vi "Insight_WL-OptFreq_Converter.vi"(6 "Units":T1(ring), 8 "error in (no error)":errorcluster, 11 "WL or Opt. Freq":dbl[](array[numeric])) -> (0 "error out":errorcluster, 3 "Opt. Freq or WL":dbl[](array[numeric]))   [LabVIEW 2010]
doc: "Insight Photonic Solutions\n\nThis VI converts wavelength to optical frequency, and vice-versa. Just input one, and the VI produces the other. Select units for wavelength and frequency.\n\nINPUTS\n\nUnits - for wavelength (nm, microns) and optical frequency (GHz, THz)\nWL or Opt. Freq - 1d array containing the input wavelength or optical frequency\nerror in - LabView error cluster\n\nOUTPUTS\nOpt. Freq. or WL - 1d array containing the calculated optical frequency or wavelength\nerror out - LabView error cluster. This is a pass-through.\n\nver 1.0 - original release"
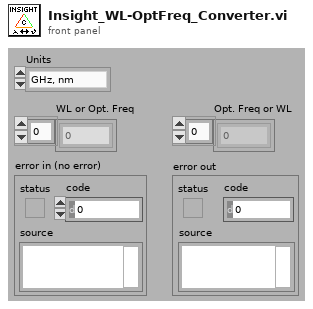
[diagram p1: front panel]
types:
  T1 = enum16{"GHz, nm", "GHz, microns", "THz, nm", "THz, microns"}
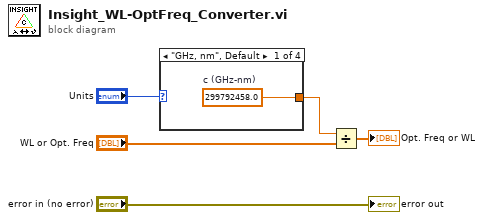
[diagram p0: block diagram]
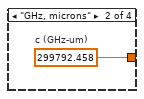
[diagram p2: hidden frame]
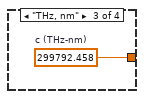
[diagram p3: hidden frame]
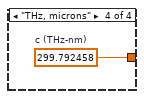
[diagram p4: hidden frame]
diagram:
  n1 = case shown="\"GHz, nm\", Default" "Units" {
    tunnel: [w6 w7 w8 w9] -> w2
    frame "GHz, nm", Default {
      w6 = 299792458.0  # c (GHz-nm)
    }
    frame "GHz, microns" {
      w7 = 299792.458  # c (GHz-um)
    }
    frame "THz, nm" {
      w8 = 299792.458  # c (THz-nm)
    }
    frame "THz, microns" {
      w9 = 299.792458  # c (THz-nm)
    }
  }
  n2 = Divide(x=w2, y="WL or Opt. Freq") -> (x/y=→"Opt. Freq or WL":dbl[])
  "error out" <- "error in (no error)"
